vi "ParseHeaderParameter.vi"(8 "default value":string, 10 "property":string, 11 "header":string) -> (3 "value":string)   [LabVIEW 2020]
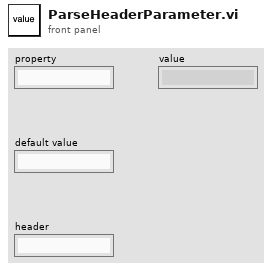
[diagram p1: front panel]
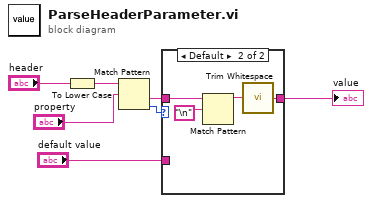
[diagram p0: block diagram]
diagram:
  n1 = To Lower Case(string="header") -> (all lower case string=w5:string)
  n2 = Match Pattern(string=w5, regular expression="property") -> (after substring=w1:string, offset past match=w2:i32)  [unwired: 1 in, 2 out]
  n3 = case shown="Default" w2 {
    tunnel: w1 -> [_ w11]
    tunnel: [w8 w12] -> w7
    tunnel: "default value" -> [w8 _]
    frame -1 {
    }
    frame Default {
      n4 = Match Pattern(string=w11, regular expression="\n") -> (before substring=w10:string)  [unwired: 1 in, 3 out]
      n5 = call <vilib>:"Trim Whitespace.vi"("string"=w10) -> ("trimmed string"=w12:string)  [unwired: 1 in]
    }
  }
  "value" <- w7
